vi "Initialize Sink.vi"(11 "Buffered Log Sink in":refnum<class "Buffered Log Sink.lvclass">) -> (0 "error out":errorcluster, 3 "Buffered Log Sink out":refnum<class "Buffered Log Sink.lvclass">)   [LabVIEW 2019, in "Buffered Log Sink.lvclass"]
uses:
  Buffered Log Sink.lvclass
  Buffered Log Sink.lvclass/Buffered Log Sink.ctl
  Composed Log/Log Sink/Log Sink.lvclass
  Composed Log/Types/Log Packet.ctl
  Composed Log/Types/Log Level.ctl
  Timeout Watchdog.vi
  Composed Log/Composed Log.lvlib
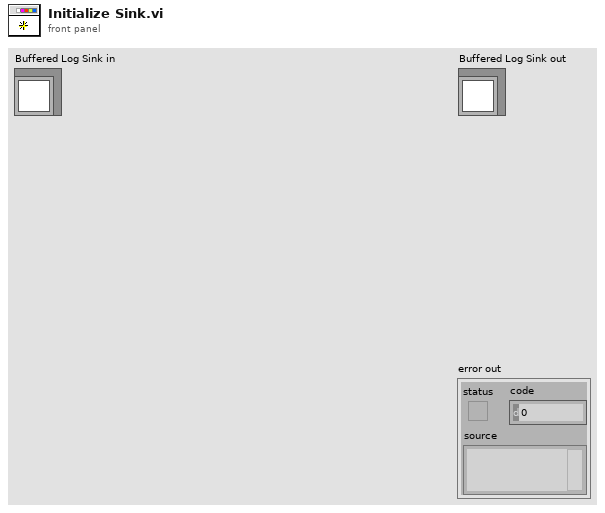
[diagram p1: front panel]
types:
  T1 = typedef "Composed Log.lvlib/Log Packet.ctl" = cluster{"Data To Log":string, "Source":string, "Event Level":T2, "Event Time":timestamp}
  T2 = typedef "Composed Log.lvlib/Log Level.ctl" = enum16{"Debug", "Info", "Warning", "Error", "Critical"}
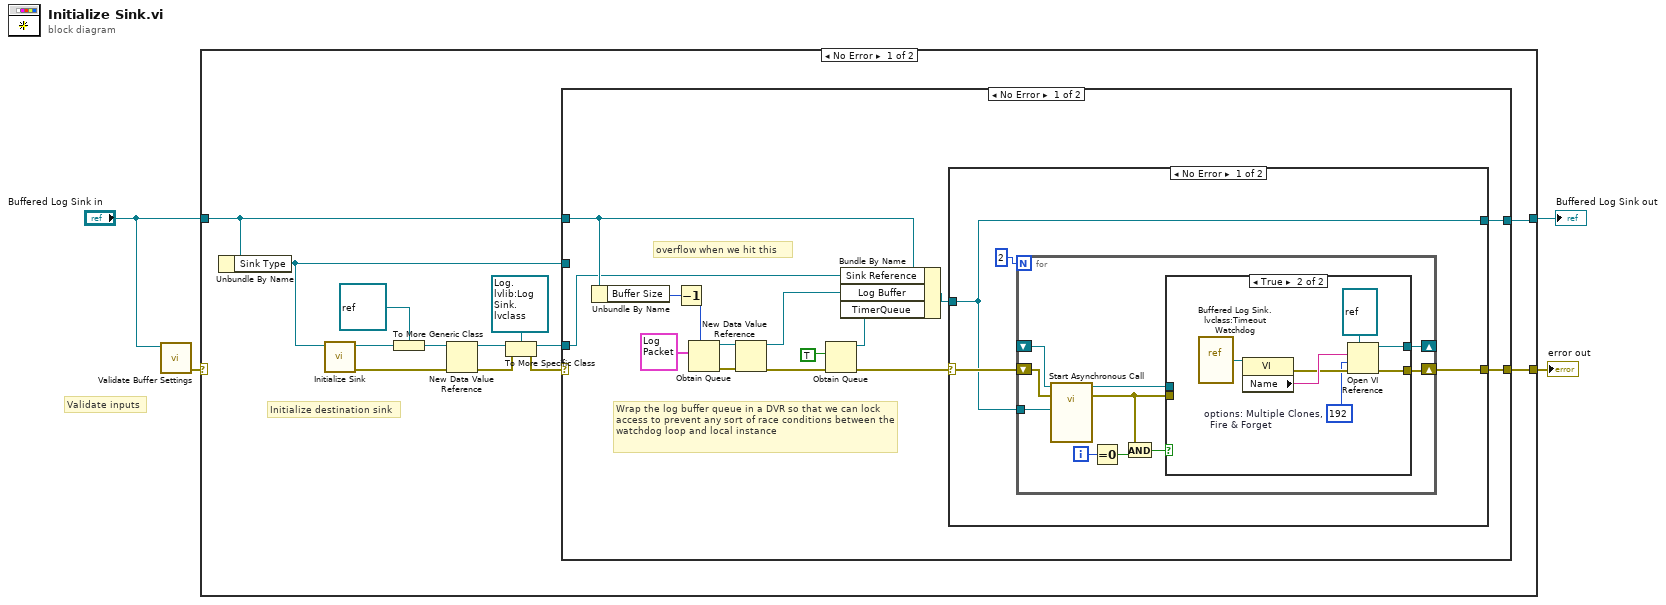
[diagram p0: block diagram]
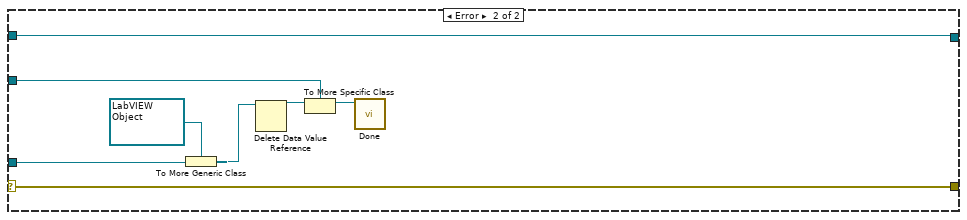
[diagram p4: hidden frame]
diagram:
  # "Validate inputs"
  n1 = call "Validate Buffer Settings.vi"("Buffered Log Sink in"="Buffered Log Sink in") -> ("error out"=w1:errorcluster)  [unwired: 10 in]
  n2 = case shown="No Error" w1 {
    selector: w1 -> [_ w66]
    tunnel: [w17 w67] -> w4
    tunnel: [w16 w66] -> w3
    tunnel: "Buffered Log Sink in" -> [w12 w67]
    frame No Error {
      # "Initialize destination sink"
      n3 = Unbundle By Name(w12) -> ("Sink Type"=w10:refnum<class "Log Sink.lvclass">)
      n4 = call-dynamic "Initialize Sink.vi"("Log Sink in"=w10) -> ("error out"=w11:errorcluster, "Log Sink out"=w15:refnum<class "Log Sink.lvclass">)  [unwired: 9 in]
      n5 = To More Generic Class(target class=refnum<class> refnum ("LabVIEW Object"), reference=w15) -> (generic class reference=w13:refnum<class>)
      n6 = New Data Value Reference(data value=w13, error in=w11) -> (data value reference=w9:refnum<data-value>, error out=w7:errorcluster)
      n7 = To More Specific Class(target class=refnum<data-value> refnum ("Sink Reference"), reference=w9, error in=w7) -> (specific class reference=w5:refnum<data-value>, error out=w6:errorcluster)
      n8 = case shown="No Error" w6 {
        selector: w6 -> [_ w64]
        tunnel: [w22 w65] -> w17
        tunnel: [w21 w64] -> w16
        tunnel: w12 -> [w20 w65]
        tunnel: w5 -> [w19 w61]
        tunnel: w10 -> [_ w63]
        frame No Error {
          # "overflow when we hit this"
          # "Wrap the log buffer queue in a DVR so that we can lock access to prevent any sort of race conditions between the watchdog loop and local instance"
          n9 = Unbundle By Name(w20) -> ("Buffer Size"=w26:i32)
          n10 = Decrement(x=w26) -> (x-1=w18:i32)
          n11 = Obtain Queue(max queue size (-1, unlimited)=w18, element data type=T1 {"Data To Log"="", "Source"="", "Event Level"=enum."Debug", "Event Time"=timestamp(0 s since 1904-01-01)} ("Log Packet")) -> (queue out=w28:refnum<queue>, error out=w25:errorcluster)  [unwired: 3 in, 1 out]
          n12 = New Data Value Reference(data value=w28, error in=w25) -> (data value reference=w27:refnum<data-value>, error out=w24:errorcluster)
          n13 = Obtain Queue(element data type=TRUE, error in (no error)=w24) -> (queue out=w29:refnum<queue>, error out=w23:errorcluster)  [unwired: 3 in, 1 out]
          n14 = Bundle By Name(cluster=w20, "Sink Reference"=w19, "Log Buffer"=w27, "TimerQueue"=w29) -> (w30:refnum<class "Buffered Log Sink.lvclass">)
          n15 = case shown="No Error" w23 {
            selector: w23 -> [w35 w56]
            tunnel: w30 -> [w34 w57]
            tunnel: [w34 w57] -> w22
            tunnel: [w33 w56] -> w21
            frame No Error {
              n16 = for {
                N: 2 -> [_]
                shift-right: [w42] -> _
                shift-left: _ -> [w46]
                tunnel: w34 -> [w38]
                shift-right: [w40] -> w33
                shift-left: w35 -> [w37]
                i -> [w45]
                n17 = call-by-ref "Start Asynchronous Call"(reference=w46, error in=w37, "Buffered Log Sink in"=w38) -> (reference out=w43:refnum<vi>, error out=w39:errorcluster)  [unwired: 11 in]
                n18 = Equal To 0?(x=w45) -> (x = 0?=w44:bool)
                n19 = And(x=w39, y=w44) -> (x .and. y?=w41:bool)
                n20 = case shown="True" w41 {
                  tunnel: w43 -> [w48 _]
                  tunnel: [w47 w51] -> w40
                  tunnel: [w48 w50] -> w42
                  tunnel: w39 -> [w47 _]
                  frame False {
                  }
                  frame True {
                    w49 = 192  # options: Multiple Clones,   Fire & Forget
                    n21 = vi-ref "Buffered Log Sink.lvclass:Timeout Watchdog.vi"() -> (w53:refnum<vi>)
                    n22 = property class="VI"(reference=w53) -> (error out=w54:errorcluster, "Name"=w55:string)  [unwired: 1 in, 1 out]
                    n23 = Open VI Reference(type specifier VI Refnum (for type only)=refnum<vi> refnum, vi path=w55, options=w49, error in (no error)=w54) -> (vi reference=w50:refnum<vi>, error out=w51:errorcluster)  [unwired: 2 in]
                  }
                }
              }
            }
            frame Error {
            }
          }
        }
        frame Error {
          n24 = To More Generic Class(target class=refnum<data-value> refnum ("data value reference"), reference=w61) -> (generic class reference=w59:refnum<data-value>)
          n25 = Delete Data Value Reference(data value reference=w59) -> (data value=w58:refnum<class>)  [unwired: 1 in, 1 out]
          n26 = To More Specific Class(target class=w63, reference=w58) -> (specific class reference=w62:refnum<class "Log Sink.lvclass">)  [unwired: 1 in, 1 out]
          n27 = call-dynamic "Done.vi"("Log Sink in"=w62) -> ()  [unwired: 10 in, 1 out]
        }
      }
    }
    frame Error {
      # "Invalid buffer settings"
    }
  }
  "error out" <- w3
  "Buffered Log Sink out" <- w4
